vi "svfa_Build Spectrum Info (N pairs) (Dual).vi"(0 "stimulus signals X [EUx]":waveform(dbl)[](array[waveform]), 1 "processing control":T7(ring), 5 "response signals Y [EUy]":waveform(dbl)[](array[waveform]), 7 "window":T8=1 items=["None"=0, "Hanning"=1, "Hamming"=2, "Blackman-Harris"=3, "Exact Blackman"=4, "Blackman"=5, "Flat Top"=6, "4 Term B-Harris "=7, "7 Term B-Harris"=8, "Low Sidelobe"=9, "Force - Exponential"=10, "Blackman Nuttall"=11, "Triangle"=30, "Bartlett-Hanning"=31, "Bohman"=32, "Parzen"=33, "Welch"=34, "Kaiser"=60, "Dolph-Chebyshev"=61, "Gaussian"=62], 9 "window size":i32, 11 "error in (no error)":errorcluster, 12 "spectrum type":T3=enum."Frequency Response [Complex]", 13 "x-axis units":u16(ring)=1 items=["time"=0, "frequency"=1, "quefrency"=2, "revolutions"=3, "order"=4, "rpm"=11], 14 "spectra info in":T1[](array[typedef]) {"x-axis units" items=["Time (s)"=0, "Frequency-CB (Hz)"=1, "Frequency-CPB (Hz)"=1248, "Frequency-Arbitrary (Hz)"=2357, "Quefrency (s)"=2, "Revolutions (rev)"=3, "Order"=4, "Speed (RPM)"=11, "Speed (rad/s)"=21, "Index"=65535]; "weighting filter" items=["Linear", "A-weighting", "B-weighting", "C-weighting", "ITU-R 468-4", "Dolby", "CCITT", "C-message", "Wb", "Wc", "Wd", "We", "Wf", "Wh", "Wj", "Wk", "Wm", "AES17 20 kHz lowpass", "AES17 40 kHz lowpass", "AES17 20 kHz highpass", "AES17 40 kHz highpass"]; "dB reference [EU]" format="%.2f"; "engineering units" items=["custom..."=0, "V"=1, "A"=21, "C"=30, "pC"=31, "s"=32, "-"=29, "Pa"=2, "N"=20, "g"=3, "m/s^2"=4, "m/s"=5, "m"=6, "mm/s"=12, "mm"=13, "micron/s"=14, "micron"=15, "in/s^2"=7, "in/s"=8, "in"=9, "mil/s"=10, "mil"=11, "rad/s^2"=16, "rad/s"=17, "rad"=18, "deg/s^2"=26, "deg/s"=27, "deg"=28, "RPM"=22, "cycle/s^2"=23, "Hz"=24, "cycle"=25, "strain"=19]; "spectral info"."window" items=["None "=0, "Hanning"=1, "Hamming"=2, "Blackman-Harris"=3, "Exact Blackman"=4, "Blackman"=5, "Flat Top"=6, "4 Term B-Harris "=7, "7 Term B-Harris"=8, "Low Sidelobe"=9, "Force - Exponential"=10, "Gaussian"=62]}) -> (3 "dup processing control":T7(ring), 4 "dup stimulus signals X [EUx]":waveform(dbl)[](array[waveform]), 6 "response signals Y [EUy]":waveform(dbl)[](array[waveform]), 10 "spectra info out":T1[](array[typedef]) {"x-axis units" items=["Time (s)"=0, "Frequency-CB (Hz)"=1, "Frequency-CPB (Hz)"=1248, "Frequency-Arbitrary (Hz)"=2357, "Quefrency (s)"=2, "Revolutions (rev)"=3, "Order"=4, "Speed (RPM)"=11, "Speed (rad/s)"=21, "Index"=65535]; "weighting filter" items=["Linear", "A-weighting", "B-weighting", "C-weighting", "ITU-R 468-4", "Dolby", "CCITT", "C-message", "Wb", "Wc", "Wd", "We", "Wf", "Wh", "Wj", "Wk", "Wm", "AES17 20 kHz lowpass", "AES17 40 kHz lowpass", "AES17 20 kHz highpass", "AES17 40 kHz highpass"]; "dB reference [EU]" format="%.2f"; "engineering units" items=["custom..."=0, "V"=1, "A"=21, "C"=30, "pC"=31, "s"=32, "-"=29, "Pa"=2, "N"=20, "g"=3, "m/s^2"=4, "m/s"=5, "m"=6, "mm/s"=12, "mm"=13, "micron/s"=14, "micron"=15, "in/s^2"=7, "in/s"=8, "in"=9, "mil/s"=10, "mil"=11, "rad/s^2"=16, "rad/s"=17, "rad"=18, "deg/s^2"=26, "deg/s"=27, "deg"=28, "RPM"=22, "cycle/s^2"=23, "Hz"=24, "cycle"=25, "strain"=19]; "spectral info"."window" items=["None "=0, "Hanning"=1, "Hamming"=2, "Blackman-Harris"=3, "Exact Blackman"=4, "Blackman"=5, "Flat Top"=6, "4 Term B-Harris "=7, "7 Term B-Harris"=8, "Low Sidelobe"=9, "Force - Exponential"=10, "Gaussian"=62]}, 15 "error out":errorcluster)   [LabVIEW 2017]
uses:
  <vilib>/addons/_NISVFA/_Shared subVIs/Controls/svc_Spectrum Info.ctl
  <vilib>/addons/_NISVFA/_Shared subVIs/Controls/svc_X-Axis Units.ctl
  <vilib>/addons/_NISVFA/_Shared subVIs/Controls/svc_Spectrum Type.ctl
  <vilib>/addons/_NISVFA/_Shared subVIs/Controls/svc_Engineering Units Text Ring.ctl
  <vilib>/addons/_NISVFA/_Shared subVIs/Controls/svc_Weighting Filter Text Ring.ctl
  <vilib>/addons/_NISVFA/_Shared subVIs/Controls/svc_Complimentary Spectrum Units.ctl
  <vilib>/addons/_NISVFA/_Shared subVIs/Controls/svc_Window [Dual FFT].ctl
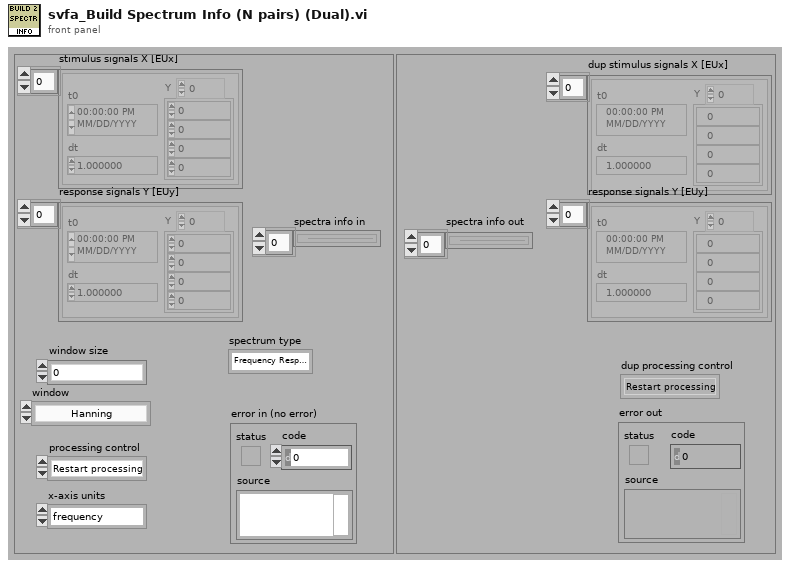
[diagram p1: front panel]
types:
  T1 = typedef "svc_Spectrum Info.ctl" = cluster{"channel name":string, "description":string, "x-axis units":T2, "spectral info":cluster{"spectrum type":T3, "linear/dB":enum16{"linear", "dB"}, "window":u16, "window size":i32, "FFT size":i32}, "engineering units":T4, "custom label":string, "dB reference [EU]":dbl, "peak units":enum16{"rms", "peak", "peak-peak"}, "weighting filter":T5, "spectral density?":bool, "unit label":string, "spectrum skewed?":bool, "complimentary spectrum units":T6}
  T2 = typedef "svc_X-Axis Units.ctl" = u16
  T3 = typedef "svc_Spectrum Type.ctl" = enum16{"FFT Spectrum [complex]", "Amplitude [Magnitude]", "Power [Magnitude^2]", "Cross Spectrum [complex]", "Frequency Response [Complex]"}
  T4 = typedef "svc_Engineering Units Text Ring.ctl" = u16
  T5 = typedef "svc_Weighting Filter Text Ring.ctl" = u16
  T6 = typedef "svc_Complimentary Spectrum Units.ctl" = enum16{"none", "radians", "degrees", "cycles", "imaginary"}
  T7 = enum16{"Restart processing", "Continue processing", "Skip processing"}
  T8 = typedef "svc_Window [Dual FFT].ctl" = u32
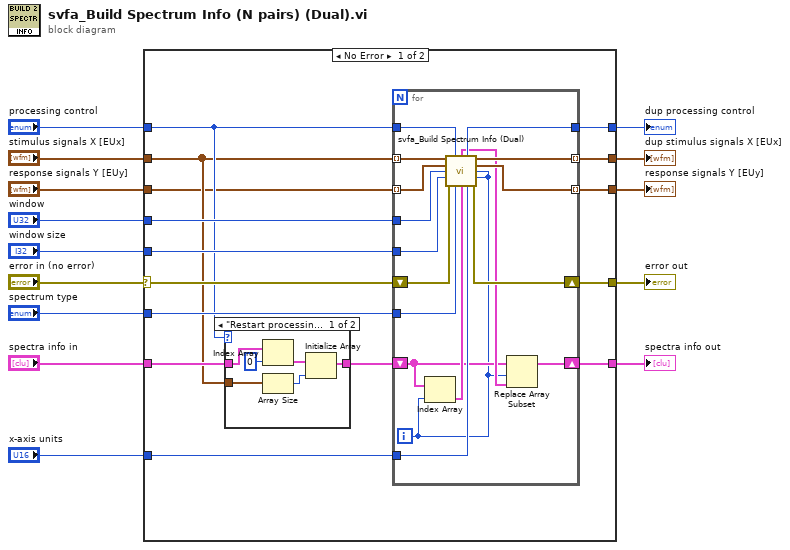
[diagram p0: block diagram]
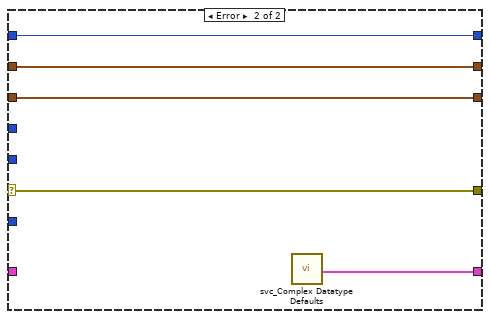
[diagram p3: hidden frame]
diagram:
  n1 = case shown="No Error" "error in (no error)" {
    selector: "error in (no error)" -> [w26 w58]
    tunnel: [w21 w54] -> w3
    tunnel: "stimulus signals X [EUx]" -> [w16 w57]
    tunnel: [w29 w57] -> w7
    tunnel: [w25 w58] -> w13
    tunnel: "response signals Y [EUy]" -> [w15 w56]
    tunnel: [w28 w56] -> w6
    tunnel: "spectrum type" -> [w27 _]
    tunnel: "window" -> [w24 _]
    tunnel: "window size" -> [w23 _]
    tunnel: "processing control" -> [w19 w55]
    tunnel: [w22 w55] -> w5
    tunnel: "spectra info in" -> [w18 _]
    tunnel: "x-axis units" -> [w20 _]
    frame No Error {
      n2 = case shown="\"Restart processing\"" w19 {
        tunnel: [w51 w53] -> w17
        tunnel: w18 -> [w52 w53]
        tunnel: w16 -> [w48 _]
        frame "Restart processing" {
          n3 = Index Array(array=w52, index=0 ("index (row)")) -> (element=w50:T1)
          n4 = Array Size(array=w48) -> (size(s)=w47:i32)
          n5 = Initialize Array(w50, w47) -> (w51:T1[])
        }
        frame "Continue processing", Default {
        }
      }
      n6 = for {
        tunnel: w16 -> [w43] mode=indexing
        tunnel: [w41] -> w29 mode=indexing
        tunnel: w15 -> [w44] mode=indexing
        tunnel: [w40] -> w28 mode=indexing
        tunnel: w27 -> [w42]
        tunnel: w24 -> [w46]
        tunnel: w23 -> [w45]
        tunnel: w19 -> [w39]
        tunnel: [w38] -> w22
        shift-right: [w36] -> w25
        shift-left: w26 -> [w37]
        tunnel: w20 -> [w35]
        shift-right: [w31] -> w21
        shift-left: w17 -> [w32]
        i -> [w30]
        n7 = Index Array(array=w32, index=w30) -> (element=w34:T1)
        n8 = call <vilib>:"svfa_Build Spectrum Info (Dual).vi"("scaled signal  X [EU]"=w43, "processing control"=w39, "scaled signal  Y [EU]"=w44, "window"=w46, "x-channel index"=w30, "window size"=w45, "y-channel index"=w30, "error in (no error)"=w37, "spectrum type"=w42, "spectrum info in"=w34, "x-axis units"=w35) -> ("spectrum info out"=w33:T1, "dup processing control"=w38:T7, "dup scaled signal  X [EU]"=w41:waveform(dbl), "dup scaled signal  Y [EU]"=w40:waveform(dbl), "error out"=w36:errorcluster)
        n9 = Replace Array Subset(array=w32, new element=w33, index=w30) -> (w31:T1[])
      }
    }
    frame Error {
      n10 = call <vilib>:"svc_Complex Datatype Defaults.vi"() -> ("empty array of spectrum info"=w54:T1[])  [unwired: 11 in, 8 out]
    }
  }
  "spectra info out" <- w3
  "error out" <- w13
  "dup processing control" <- w5
  "dup stimulus signals X [EUx]" <- w7
  "response signals Y [EUy]" <- w6
